vi "Testing Rendevous Abort.vi"() -> ()   [LabVIEW 2021]
panel:
  out "error out 2":errorcluster
  out "error out":errorcluster
  in  "stop":bool
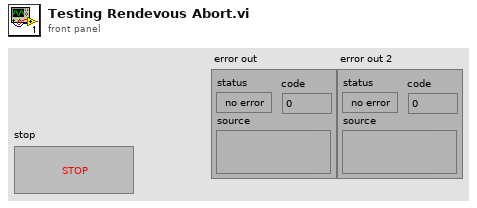
[diagram p1: front panel]
types:
  T1 = typedef "Rendezvous RefNum" = refnum<k1>
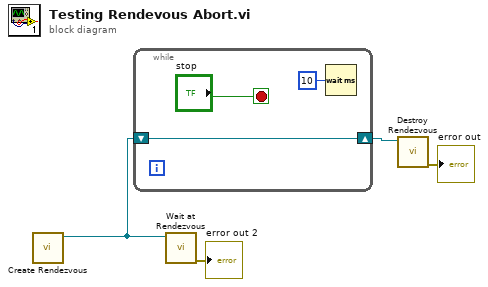
[diagram p0: block diagram]
diagram:
  n1 = call <vilib>:"Create Rendezvous.vi"() -> ("rendezvous"=w4:T1)  [unwired: 5 in, 2 out]
  n2 = while {
    shift-right: [w5] -> w3
    shift-left: w4 -> [w5]
    stop <- "stop" stop-if-true
    n3 = Wait (ms)(milliseconds to wait=u32 10) -> ()  [unwired: 1 out]
  }
  n4 = call <vilib>:"Wait at Rendezvous.vi"("rendezvous"=w4) -> ("error out"=→"error out 2":errorcluster)  [unwired: 4 in, 2 out]
  n5 = call <vilib>:"Destroy Rendezvous.vi"("rendezvous"=w3) -> ("error out"=→"error out":errorcluster)  [unwired: 5 in, 1 out]
